vi "delta_k.vi"(10 "Expected Output":dbl, 11 "Output":dbl) -> (3 "Delta K":dbl[](array[numeric]))   [LabVIEW 2018]
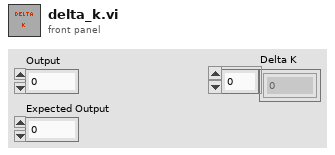
[diagram p1: front panel]
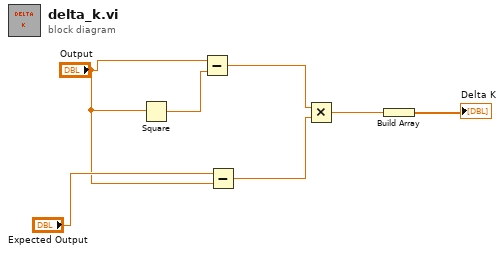
[diagram p0: block diagram]
diagram:
  n1 = Square(x="Output") -> (x^2=w7:dbl)
  n2 = Subtract(x="Output", y=w7) -> (x-y=w6:dbl)
  n3 = Subtract(x="Expected Output", y="Output") -> (x-y=w5:dbl)
  n4 = Multiply(x=w6, y=w5) -> (x*y=w2:dbl)
  n5 = Build Array(w2) -> (→"Delta K":dbl[])
